vi "ComunicaciónSerial_Posición.vi"() -> ()   [LabVIEW 2023]
uses:
  <vilib>/Instr/_visa.llb/VISA Configure Serial Port (Instr).vi
panel:
  out "Grados forma 2":dbl(knob) scale=0.0..360.0
  out "Grados":dbl
  in  "baud rate":u32=9600
  out "Grados forma 1":dbl(knob) scale=0.0..360.0
  in  "Set Point":dbl
  in  "Mandar datos":bool
  in  "byte count":u32
  in  "VISA resource name":refnum<visa-resource-name>
  in  "stop":bool
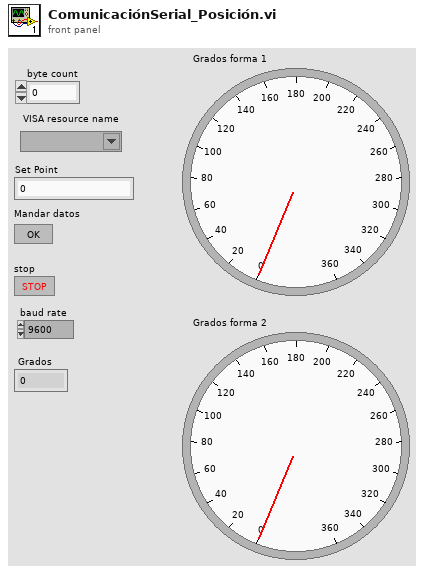
[diagram p1: front panel]
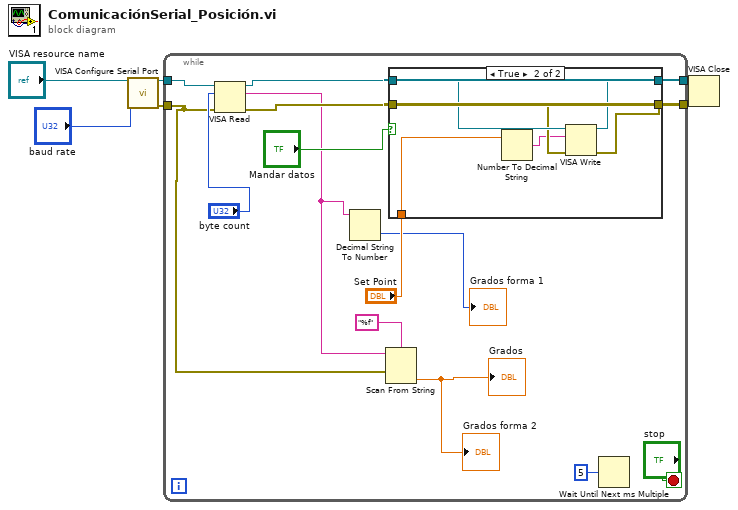
[diagram p0: block diagram]
diagram:
  n1 = call-poly "VISA Configure Serial Port"("VISA resource name"="VISA resource name", "baud rate (9600)"="baud rate") -> ("VISA resource name out"=w5:refnum<visa-resource-name>, "error out"=w6:errorcluster)  [unwired: 12 in]
  n2 = while {
    tunnel: w6 -> [w9]
    tunnel: w5 -> [w17]
    tunnel: [w15] -> w4
    tunnel: [w14] -> w3
    stop <- "stop" stop-if-true
    n3 = VISA Read(VISA resource name=w17, byte count="byte count", error in (no error)=w9) -> (VISA resource name out=w15:refnum<visa-resource-name>, read buffer=w10:string, error out=w14:errorcluster)  [unwired: 1 out]
    n4 = Decimal String To Number(string=w10) -> (number=→"Grados forma 1":i32)  [unwired: 2 in, 1 out]
    n5 = Scan From String(format string="%f", input string=w10, error in=w9) -> (output 1=→"Grados" →"Grados forma 2":dbl)  [unwired: 2 in, 3 out]
    n6 = case shown="True" "Mandar datos" {
      tunnel: w15 -> [w21 w27]
      tunnel: w14 -> [w20 w26]
      tunnel: [w21 w23] -> _
      tunnel: [w20 w22] -> _
      tunnel: "Set Point" -> [_ w25]
      frame False {
      }
      frame True {
        n7 = Number To Decimal String(number=w25) -> (decimal integer string=w24:string)  [unwired: 1 in]
        n8 = VISA Write(VISA resource name=w27, write buffer=w24, error in (no error)=w26) -> (VISA resource name out=w23:refnum<visa-resource-name>, error out=w22:errorcluster)  [unwired: 1 out]
      }
    }
    n9 = Wait Until Next ms Multiple(millisecond multiple=u32 5) -> ()  [unwired: 1 out]
  }
  n10 = VISA Close(VISA resource name=w4, error in (no error)=w3) -> ()  [unwired: 1 out]
